vi "Get stack info.vi"(8 "error in (no error)":errorcluster, 11 "Tomo in":refnum<class "Tomo.lvclass">) -> (0 "error out":errorcluster, 1 "Z start":dbl, 2 "Z stop":dbl, 3 "Tomo out":refnum<class "Tomo.lvclass">, 4 "Y position":dbl, 5 "X position":dbl, 6 "Default focus":dbl[unit])   [LabVIEW 2012, in "Tomo.lvclass"]
uses:
  Tomo.lvclass
  Tomo.lvclass/Tomo.ctl
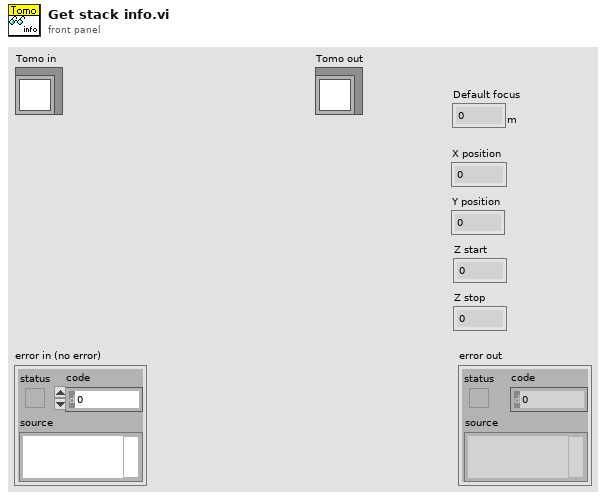
[diagram p1: front panel]
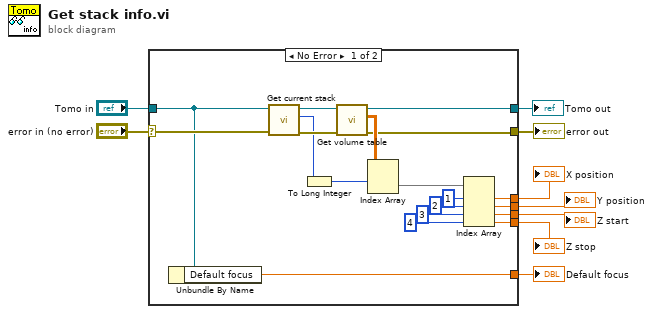
[diagram p0: block diagram]
diagram:
  n1 = case shown="No Error" "error in (no error)" {
    selector: "error in (no error)" -> [w26 w30]
    tunnel: [w17 w30] -> w8
    tunnel: [w16 w29] -> w2
    tunnel: "Tomo in" -> [w11 w29]
    tunnel: [w15 _] -> w7
    tunnel: [w14 _] -> w6
    tunnel: [w13 _] -> w5
    tunnel: [w12 _] -> w4
    tunnel: [w10 _] -> w1
    frame No Error {
      n2 = Unbundle By Name(w11) -> ("Default focus"=w10:dbl[unit])
      n3 = call-dynamic "Get current stack.vi"("error in (no error)"=w26, "Tomo in"=w11) -> ("error out"=w27:errorcluster, "Current stack"=w24:u16, "Tomo out"=w28:refnum<class "Tomo.lvclass">)  [unwired: 7 in]
      n4 = To Long Integer(number=w24) -> (32bit integer=w23:i32)
      n5 = call-dynamic "Get volume table.vi"("error in (no error)"=w27, "Tomo in"=w28) -> ("error out"=w17:errorcluster, "Volume table out"=w25:dbl[][], "Tomo out"=w16:refnum<class "Tomo.lvclass">)  [unwired: 7 in]
      n6 = Index Array(array=w25, index (row)=w23) -> (element=w22:dbl[])  [unwired: 1 in]
      n7 = Index Array(array=w22, index #1=1 ("index"), index #2=2 ("index"), index #3=3 ("index"), index #4=4 ("index")) -> (element #1=w15:dbl, element #2=w14:dbl, element #3=w13:dbl, element #4=w12:dbl)
    }
    frame Error {
    }
  }
  "error out" <- w8
  "X position" <- w7
  "Z start" <- w5
  "Y position" <- w6
  "Z stop" <- w4
  "Tomo out" <- w2
  "Default focus" <- w1
